vi "GenerateURL.vi"(7 "host":string="10.2.64.27", 8 "error in (no error)":errorcluster, 9 "port":string="8001", 10 "data":string, 11 "method":string) -> (0 "error out":errorcluster, 3 "url":string)   [LabVIEW 2017]
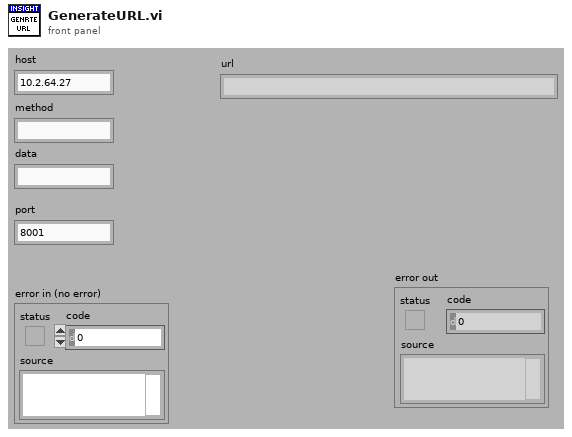
[diagram p1: front panel]
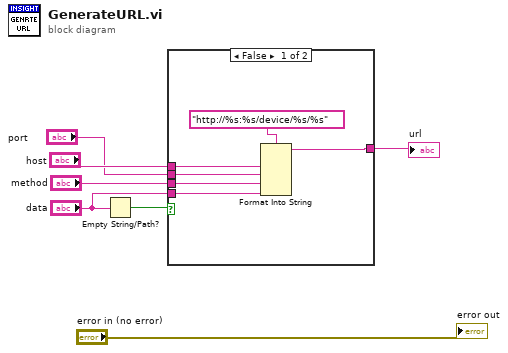
[diagram p0: block diagram]
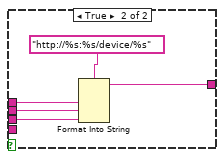
[diagram p2: hidden frame]
diagram:
  n1 = Empty String/Path?(string/path="data") -> (empty?=w7:bool)
  n2 = case shown="False" w7 {
    tunnel: "host" -> [w12 w17]
    tunnel: "method" -> [w11 w14]
    tunnel: [w9 w16] -> w4
    tunnel: "data" -> [w10 _]
    tunnel: "port" -> [w8 w15]
    frame False {
      n3 = Format Into String(format string="http://%s:%s/device/%s/%s", w12, w8, w11, w10) -> (resulting string=w9:string)  [unwired: 2 in, 1 out]
    }
    frame True {
      n4 = Format Into String(format string="http://%s:%s/device/%s", w17, w15, w14) -> (resulting string=w16:string)  [unwired: 2 in, 1 out]
    }
  }
  "url" <- w4
  "error out" <- "error in (no error)"
